vi "CSM - Run Script.vi"(0 "single-line text":string, 1 "Current Module(\"\" to generate a ID)":string, 7 "Continue If Error?(F)":bool, 9 "Wait(5000ms)":i32=5000, 11 "error in (no error)":errorcluster, 12 "Response Timeout(5000ms)":i32=5000) -> (10 "States Left":string, 15 "error out":errorcluster)   [LabVIEW 2020, in "Communicable State Machine.lvlib"]
uses:
  Communicable State Machine.lvlib
  Priority Queue.lvclass/Priority Queue.ctl
  Trim Single line Text.vi
  CSM - Wait for Module to Be Alive.vi
  CSM - Send Message and Wait for Reply.vi
  CSM - Post Message.vi
  CSM - Check If Module Exists.vi
  CSMP-Sync Call.vi
  uuid.vi
  Trim Both Whitespace.vi
  CSMP-Async Call.vi
  _Obtain CSM Data Queue.vi
  Release Priority Queue.vi
  _CSMObj-Message Check.vi
  _CSMObj-Enqueue Cross-Module Message.vi
  _CSMOFGV Get.vi
  Obtain Priority Queue.vi
  Enqueue Element.vi
  CSM No Target Error.vi
  _CSMOFGV.vi
  CSM Not Allowed Message.vi
  CSM Target Error.vi
  CSM Unhandled State Error.vi
  CSM Target Timeout Error.vi
  FGV-BroadcastRegistry.vi
  Priority Queue.lvclass
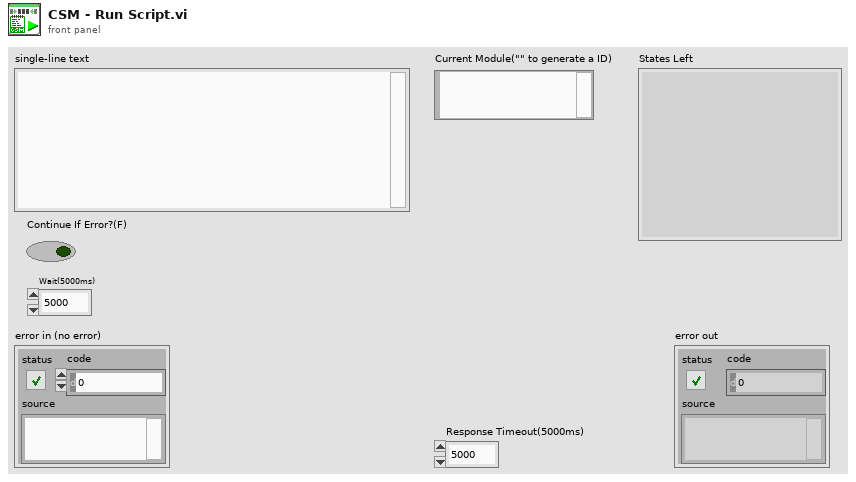
[diagram p1: front panel]
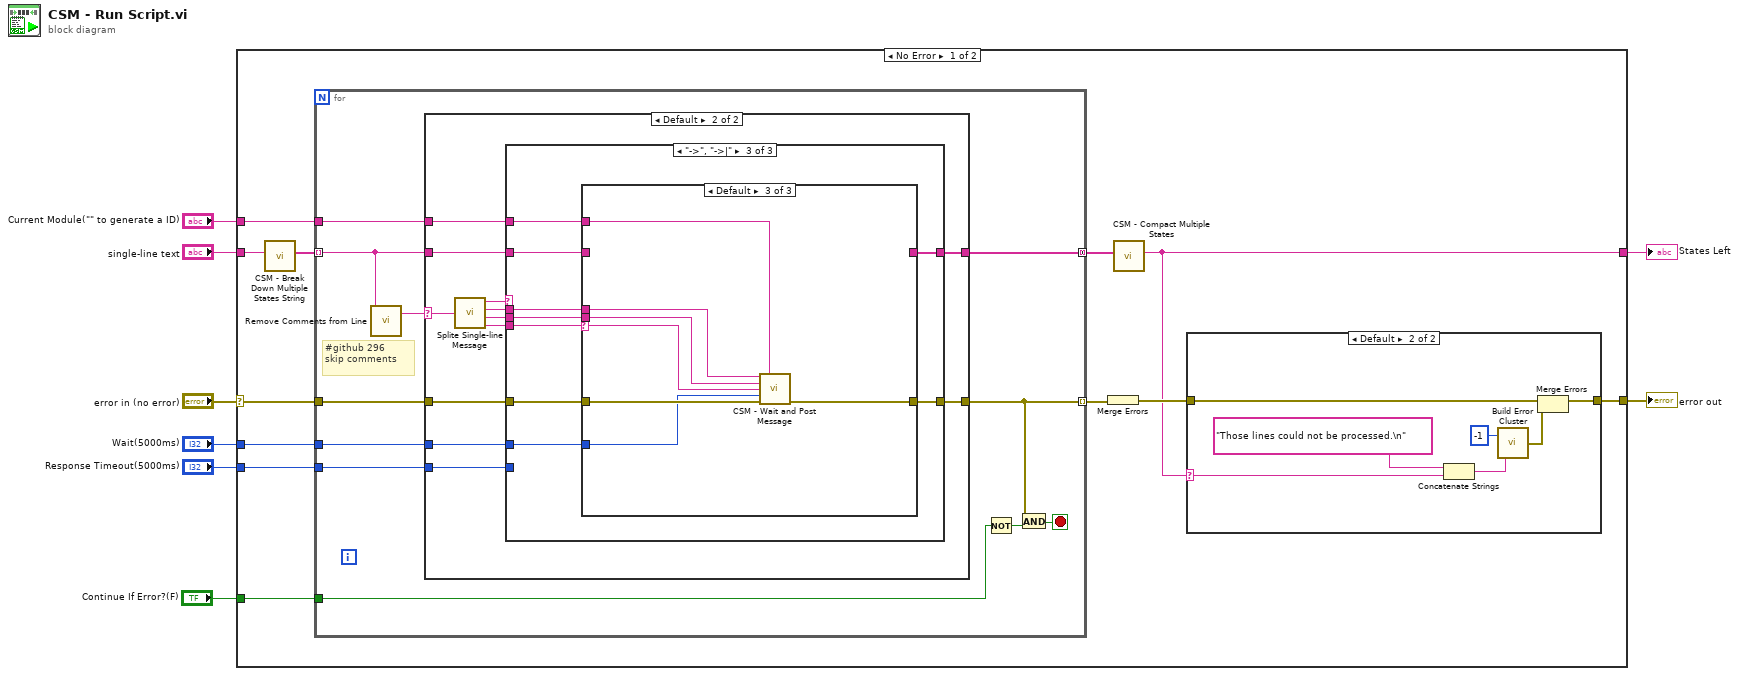
[diagram p0: block diagram]
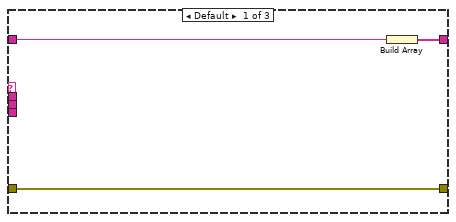
[diagram p4: hidden frame]
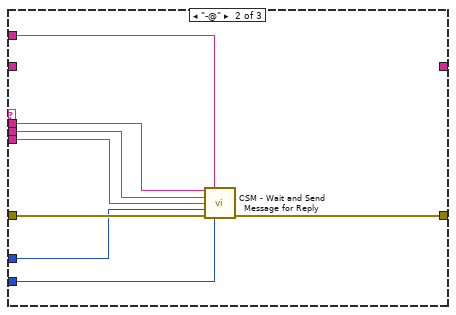
[diagram p5: hidden frame]
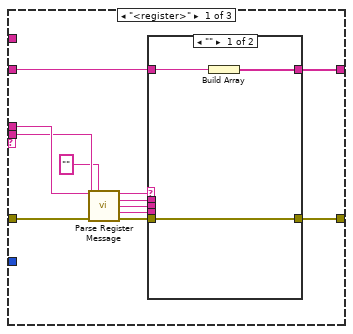
[diagram p6: hidden frame]
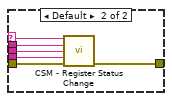
[diagram p7: hidden frame]
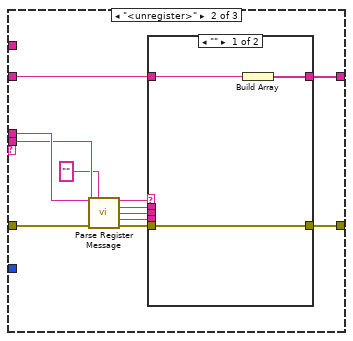
[diagram p8: hidden frame]
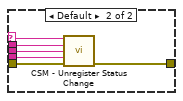
[diagram p9: hidden frame]
diagram:
  n1 = case shown="No Error" "error in (no error)" {
    selector: "error in (no error)" -> [w18 w120]
    tunnel: "single-line text" -> [w17 _]
    tunnel: [w14 _] -> w6
    tunnel: [w13 w120] -> w5
    tunnel: "Current Module(\"\" to generate a ID)" -> [w12 _]
    tunnel: "Response Timeout(5000ms)" -> [w11 _]
    tunnel: "Wait(5000ms)" -> [w10 _]
    tunnel: "Continue If Error?(F)" -> [w9 _]
    frame No Error {
      n2 = call "CSM - Break Down Multiple States String.vi"("States"=w17) -> ("Multiple States"=w16:string[])  [unwired: 10 in]
      n3 = for {
        tunnel: w16 -> [w36] mode=indexing
        tunnel: w18 -> [w39]
        tunnel: [w31] -> w19 mode=indexing
        tunnel: [w37] -> w15 mode=concatenating
        tunnel: w12 -> [w35]
        tunnel: w11 -> [w34]
        tunnel: w10 -> [w33]
        tunnel: w9 -> [w30]
        stop <- w32 stop-if-true
        # "#github 296\nskip comments"
        n4 = call "Remove Comments from Line.vi"("single-line text"=w36) -> ("single-line text without comments"=w38:string)  [unwired: 2 in]
        n5 = case shown="Default" w38 {
          selector: w38 -> [_ w46]
          tunnel: [w40 w52] -> w31
          tunnel: w39 -> [w40 w51]
          tunnel: [_ w45] -> w37
          tunnel: w36 -> [_ w44]
          tunnel: w35 -> [_ w43]
          tunnel: w34 -> [_ w42]
          tunnel: w33 -> [_ w41]
          frame "" {
          }
          frame Default {
            n6 = call "Splite Single-line Message.vi"("single-line text"=w46) -> ("operator"=w50:string, "state"=w47:string, "args"=w48:string, "source/target"=w49:string)  [unwired: 6 in]
            n7 = case shown="\"->\", \"->|\"" w50 {
              tunnel: w49 -> [_ w63 w72]
              tunnel: w48 -> [_ w62 w71]
              tunnel: w47 -> [_ w61 w70]
              tunnel: w51 -> [w55 w60 w69]
              tunnel: [w55 w59 w68] -> w52
              tunnel: [w54 _ w67] -> w45
              tunnel: w44 -> [w53 _ w66]
              tunnel: w43 -> [_ w58 w65]
              tunnel: w42 -> [_ w57 _]
              tunnel: w41 -> [_ w56 w64]
              frame Default {
                n8 = Build Array(w53) -> (w54:string[])
              }
              frame "-@" {
                n9 = call "CSM - Wait and Send Message for Reply.vi"("State"=w61, "Current Module(\"\" to generate a ID)"=w58, "Arguments (\"\")"=w62, "Target Module"=w63, "Wait(5000ms)"=w56, "Error In (no error)"=w60, "Response Timeout(5000ms)"=w57) -> ("error out"=w59:errorcluster)  [unwired: 6 in, 2 out]
              }
              frame "->", "->|" {
                n10 = case shown="Default" w72 {
                  selector: w72 -> [_ _ w119]
                  tunnel: w71 -> [w78 w98 w118]
                  tunnel: w70 -> [w79 w99 w117]
                  tunnel: w69 -> [w77 w97 w116]
                  tunnel: [w76 w96 w115] -> w68
                  tunnel: [w74 w94 _] -> w67
                  tunnel: w66 -> [w73 w93 _]
                  tunnel: w65 -> [_ _ w114]
                  tunnel: w64 -> [_ _ w113]
                  frame "<register>" {
                    n11 = call "Parse Register Message.vi"("state"=w79, "Module Name"="", "args"=w78) -> ("target"=w83:string, "source"=w82:string, "status"=w81:string, "api"=w80:string)  [unwired: 9 in]
                    n12 = case shown="\"\"" w83 {
                      selector: w83 -> [_ w92]
                      tunnel: w82 -> [_ w91]
                      tunnel: w81 -> [_ w90]
                      tunnel: w80 -> [_ w89]
                      tunnel: w77 -> [w86 w88]
                      tunnel: [w86 w87] -> w76
                      tunnel: [w84 _] -> w74
                      tunnel: w73 -> [w85 _]
                      frame "" {
                        n13 = Build Array(w85) -> (w84:string[])
                      }
                      frame Default {
                        n14 = call "CSM - Register Status Change.vi"("CSM Name"=w92, "Source CSM Name (* as Default)"=w91, "Status"=w90, "Response Message (if \"\", same as Source Message)"=w89, "Error in"=w88) -> ("Error out"=w87:errorcluster)  [unwired: 9 in, 1 out]
                      }
                    }
                  }
                  frame "<unregister>" {
                    n15 = call "Parse Register Message.vi"("state"=w99, "Module Name"="", "args"=w98) -> ("target"=w103:string, "source"=w102:string, "status"=w101:string, "api"=w100:string)  [unwired: 9 in]
                    n16 = case shown="\"\"" w103 {
                      selector: w103 -> [_ w112]
                      tunnel: w102 -> [_ w111]
                      tunnel: w101 -> [_ w110]
                      tunnel: w100 -> [_ w109]
                      tunnel: w97 -> [w106 w108]
                      tunnel: [w106 w107] -> w96
                      tunnel: [w104 _] -> w94
                      tunnel: w93 -> [w105 _]
                      frame "" {
                        n17 = Build Array(w105) -> (w104:string[])
                      }
                      frame Default {
                        n18 = call "CSM - Unregister Status Change.vi"("CSM Name"=w112, "Source CSM Name (* as Default)"=w111, "Status"=w110, "Response Message (\"*\" as Default)"=w109, "Error in"=w108) -> ("Error out"=w107:errorcluster)  [unwired: 9 in, 1 out]
                      }
                    }
                  }
                  frame Default {
                    n19 = call "CSM - Wait and Post Message.vi"("State"=w117, "Current Module(\"\" to generate a ID)"=w114, "Arguments (\"\")"=w118, "Target Module"=w119, "Wait(5000ms)"=w113, "Error In (no error)"=w116) -> ("error out"=w115:errorcluster)  [unwired: 9 in]
                  }
                }
              }
            }
          }
        }
        n20 = Not(x=w30) -> (.not. x?=w29:bool)
        n21 = And(x=w31, y=w29) -> (x .and. y?=w32:bool)
      }
      n22 = Merge Errors(w19) -> (w20:errorcluster)
      n23 = call "CSM - Compact Multiple States.vi"("Multiple States"=w15) -> ("States"=w14:string)  [unwired: 9 in]
      n24 = case shown="Default" w14 {
        selector: w14 -> [_ w24]
        tunnel: w20 -> [w21 w28]
        tunnel: [w21 w23] -> w13
        frame "" {
        }
        frame Default {
          n25 = Concatenate Strings("Those lines could not be processed.\n" ("String to Prepend to source (\"\")"), w24) -> (w25:string)
          n26 = call "Build Error Cluster.vi"("String to Prepend to source (\"\")"=w25, "code"=-1) -> ("error out"=w22:errorcluster)
          n27 = Merge Errors(w28, w22) -> (w23:errorcluster)
        }
      }
    }
    frame Error {
    }
  }
  "error out" <- w5
  "States Left" <- w6
